vi "ubinary.vi"(11 "Cluster":variant) -> (1 "Debug Timing":cluster{"Time":u32, "Data Name":string}[](array[cluster]), 3 "Header":cluster{"Element Names":string[], u8[]})   [LabVIEW 2012]
uses:
  <userlib>/_OpenG.lib/lvdata/lvdata.llb/Type Descriptor Enumeration__ogtk.ctl
panel:
  out "sum":u32
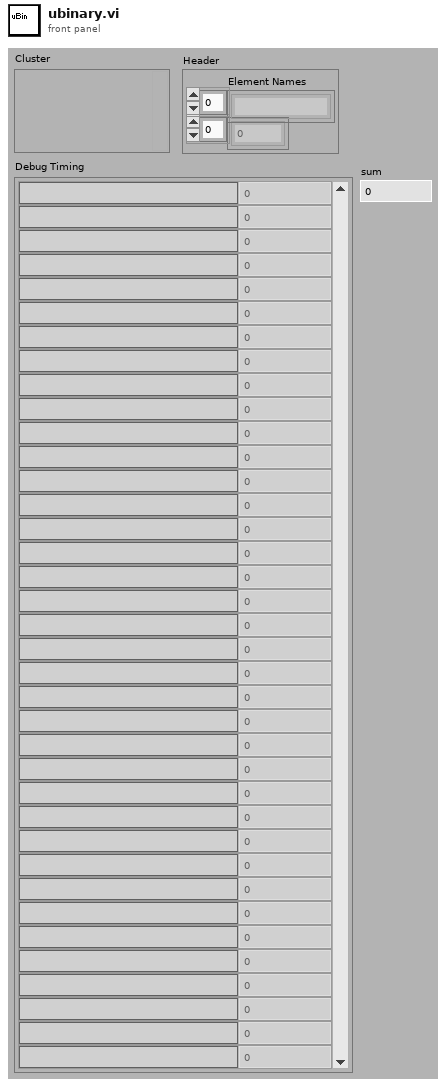
[diagram p1: front panel]
types:
  T1 = typedef "Type Descriptor Enumeration__ogtk.ctl" = enum8{"<Null>", "I8", "I16", "I32", "I64", "U8", "U16", "U32", "U64", "SGL", "DBL", "EXT", "CSG", "CDB", "CXT", "0x0F", "0x10", "0x11", "0x12", "0x13", "0x14", "Enum U8", "Enum U16", "Enum U32", "Enum U64", "SGL PQ", "DBL PQ", "EXT PQ", "CSG PQ", "CDB PQ", "CXT PQ", "0x1F", "0x20", "Boolean", "0x22", "0x23", "0x24", "0x25", "0x26", "0x27", "0x28", "0x29", "0x2A", "0x2B", "0x2C", "0x2D", "0x2E", "0x2F", "String", "0x31", "Path", "Pict", "0x34", "0x35", "0x36", "DAQ", "0x38", "0x39", "0x3A", "0x3B", "0x3C", "0x3D", "0x3E", "0x3F", "Array", "0x41", "0x42", "0x43", "0x44", "0x45", "0x46", "0x47", "0x48", "0x49", "0x4A", "0x4B", "0x4C", "0x4D", "0x4E", "0x4F", "Cluster", "0x51", "0x52", "Variant", "Waveform", "0x55", "0x56", "0x57", "0x58", "0x59", "0x5A", "0x5B", "0x5C", "0x5D", "0x5E", "0x5F", "0x60", "0x61", "0x62", "0x63", "0x64", "0x65", "0x66", "0x67", "0x68", "0x69", "0x6A", "0x6B", "0x6C", "0x6D", "0x6E", "0x6F", "Refnum"}
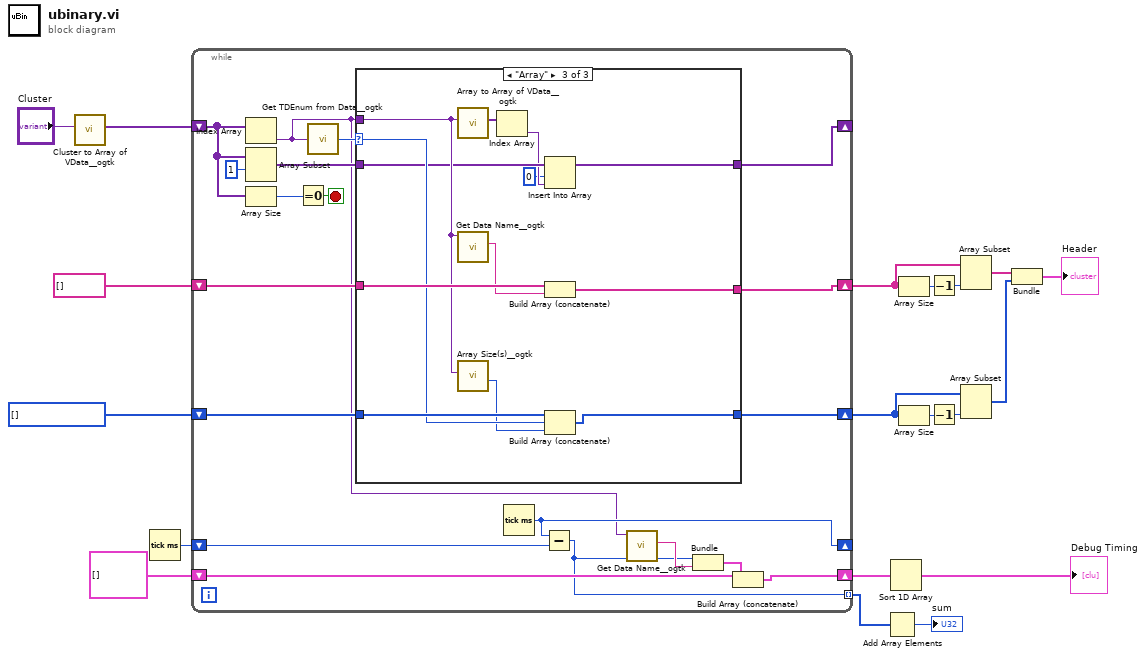
[diagram p0: block diagram]
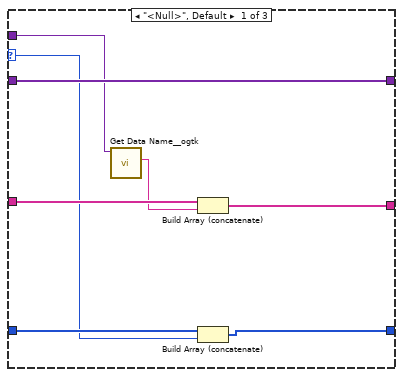
[diagram p2: hidden frame]
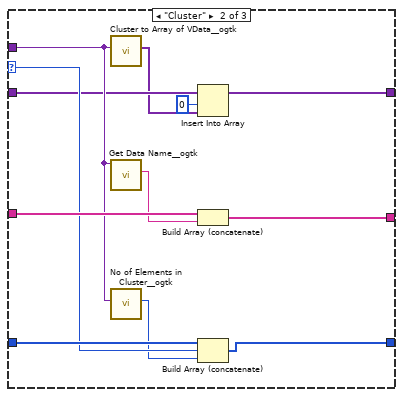
[diagram p3: hidden frame]
diagram:
  w6 = T1[] [] items=["<Null>", "I8", "I16", "I32", "I64", "U8", "U16", "U32", "U64", "SGL", "DBL", "EXT", "CSG", "CDB", "CXT", "0x0F", "0x10", "0x11", "0x12", "0x13", "0x14", "Enum U8", "Enum U16", "Enum U32", "Enum U64", "SGL PQ", "DBL PQ", "EXT PQ", "CSG PQ", "CDB PQ", "CXT PQ", "0x1F", "0x20", "Boolean", "0x22", "0x23", "0x24", "0x25", "0x26", "0x27", "0x28", "0x29", "0x2A", "0x2B", "0x2C", "0x2D", "0x2E", "0x2F", "String", "0x31", "Path", "Pict", "0x34", "0x35", "0x36", "DAQ", "0x38", "0x39", "0x3A", "0x3B", "0x3C", "0x3D", "0x3E", "0x3F", "Array", "0x41", "0x42", "0x43", "0x44", "0x45", "0x46", "0x47", "0x48", "0x49", "0x4A", "0x4B", "0x4C", "0x4D", "0x4E", "0x4F", "Cluster", "0x51", "0x52", "Variant", "Waveform", "0x55", "0x56", "0x57", "0x58", "0x59", "0x5A", "0x5B", "0x5C", "0x5D", "0x5E", "0x5F", "0x60", "0x61", "0x62", "0x63", "0x64", "0x65", "0x66", "0x67", "0x68", "0x69", "0x6A", "0x6B", "0x6C", "0x6D", "0x6E", "0x6F", "Refnum"]
  n1 = call <userlib>:"Cluster to Array of VData__ogtk.vi"("Cluster"="Cluster") -> ("Array of VData"=w18:variant[])  [unwired: 9 in, 1 out]
  n2 = Tick Count (ms)() -> (millisecond timer value=w7:u32)
  n3 = while {
    shift-right: [w37] -> _
    shift-left: w18 -> [w31]
    shift-right: [w32] -> w12
    shift-left: string[] [] -> [w35]
    shift-right: [w33] -> w13
    shift-left: w6 -> [w34]
    shift-right: [w26] -> _
    shift-left: w7 -> [w27]
    shift-right: [w23] -> w4
    shift-left: cluster{u32, "Data Name":string}[] [] -> [w22]
    tunnel: [w20] -> w2 mode=indexing
    stop <- w30 stop-if-true
    n4 = Index Array(array=w31) -> (element=w25:variant)  [unwired: 1 in]
    n5 = Array Subset(array=w31, index=1) -> (w36:variant[])  [unwired: 1 in]
    n6 = Array Size(array=w31) -> (size(s)=w28:i32)
    n7 = Equal To 0?(x=w28) -> (x = 0?=w30:bool)
    n8 = call <userlib>:"Get TDEnum from Data__ogtk.vi"("Data"=w25) -> ("Type Descriptor Enumeration"=w29:T1)  [unwired: 4 in]
    n9 = case shown="\"Array\"" w29 {
      selector: w29 -> [w41 w54 w67]
      tunnel: [w46 w49 w62] -> w37
      tunnel: w36 -> [w46 w51 w63]
      tunnel: w35 -> [w45 w58 w71]
      tunnel: w34 -> [w44 w57 w70]
      tunnel: [w43 w56 w69] -> w33
      tunnel: [w42 w55 w68] -> w32
      tunnel: w25 -> [w40 w52 w64]
      frame "<Null>", Default {
        n10 = call <userlib>:"Get Data Name__ogtk.vi"("Data"=w40) -> ("Data Name"=w39:string)  [unwired: 8 in, 2 out]
        n11 = Build Array (concatenate)(w45, w39) -> (w42:string[])
        n12 = Build Array (concatenate)(w44, w41) -> (w43:u32[])
      }
      frame "Cluster" {
        n13 = call <userlib>:"Cluster to Array of VData__ogtk.vi"("Cluster"=w52) -> ("Array of VData"=w50:variant[])  [unwired: 9 in, 1 out]
        n14 = call <userlib>:"Get Data Name__ogtk.vi"("Data"=w52) -> ("Data Name"=w47:string)  [unwired: 8 in, 2 out]
        n15 = call <userlib>:"No of Elements in Cluster__ogtk.vi"("Cluster"=w52) -> ("Number of Elements"=w53:u16)  [unwired: 9 in, 1 out]
        n16 = Insert Into Array(array=w51, index=0, new element=w50) -> (w49:variant[])
        n17 = Build Array (concatenate)(w58, w47) -> (w55:string[])
        n18 = Build Array (concatenate)(w57, w54, w53) -> (w56:u32[])
      }
      frame "Array" {
        n19 = call <userlib>:"Array to Array of VData__ogtk.vi"("MultiD Array"=w64) -> ("1D Array of Variants"=w66:variant[])  [unwired: 9 in, 1 out]
        n20 = call <userlib>:"Get Data Name__ogtk.vi"("Data"=w64) -> ("Data Name"=w59:string)  [unwired: 8 in, 2 out]
        n21 = call <userlib>:"Array Size(s)__ogtk.vi"("Array"=w64) -> ("N dims"=w65:u32)  [unwired: 8 in, 2 out]
        n22 = Index Array(array=w66) -> (element=w61:variant)  [unwired: 1 in]
        n23 = Insert Into Array(array=w63, index=0, new element=w61) -> (w62:variant[])
        n24 = Build Array (concatenate)(w71, w59) -> (w68:string[])
        n25 = Build Array (concatenate)(w70, w67, w65) -> (w69:u32[])
      }
    }
    n26 = Tick Count (ms)() -> (millisecond timer value=w26:u32)
    n27 = Subtract(x=w26, y=w27) -> (x-y=w20:u32)
    n28 = call <userlib>:"Get Data Name__ogtk.vi"("Data"=w25) -> ("Data Name"=w21:string)  [unwired: 8 in, 2 out]
    n29 = Bundle(w20, "Data Name"=w21) -> (w24:cluster{u32, "Data Name":string})  [unwired: 1 in]
    n30 = Build Array (concatenate)(w22, w24) -> (w23:cluster{u32, "Data Name":string}[])
  }
  n31 = Add Array Elements(numeric array=w2) -> (sum=→"sum":u32)
  n32 = Sort 1D Array(array=w4) -> (sorted array=→"Debug Timing":cluster{u32, "Data Name":string}[])
  n33 = Array Size(array=w12) -> (size(s)=w15:i32)
  n34 = Array Size(array=w13) -> (size(s)=w17:i32)
  n35 = Decrement(x=w15) -> (x-1=w14:i32)
  n36 = Decrement(x=w17) -> (x-1=w16:i32)
  n37 = Array Subset(array=w12, length=w14) -> (w11:string[])  [unwired: 1 in]
  n38 = Array Subset(array=w13, length=w16) -> (w10:u32[])  [unwired: 1 in]
  n39 = Bundle(w11, w10) -> (→"Header":cluster{string[], u32[]})  [unwired: 1 in]
